vi "Test Error Propagation VITester Verify.vi"(8 "error in":errorcluster, 11 "Error.Tests in":refnum<class "Error.Propagation.Tests.lvclass">) -> (0 "error out":errorcluster, 3 "Error.Tests out":refnum<class "Error.Propagation.Tests.lvclass">)   [LabVIEW 2026, in "Error.Propagation.Tests.lvclass"]
uses:
  Error.Propagation.Tests.lvclass
  Source/Approval Tests/Options/Options.lvclass
  <vilib>/Addons/_JKI Toolkits/VI Tester/TestCase.llb/TestCase.lvclass
  Source/Approval Tests/Options/Options.lvclass/Options.ctl
  Source/Approval Tests/Naming Data/Naming Data.lvclass/Naming Data.ctl
  020b3fef-1487-42c6-8763-2b116f719ab6.vi
  020b3fef-1487-42c6-8763-2b116f719ab6.vi/ef028380-787c-4fa5-86c8-b0b7860ce2dc.vi
  Source/Approval Tests/Replace if Empty.vi
  Source/Approval Tests/Update Test Name if Not Defined.vi
  Source/Approval Tests/Verify Core.vi
  020b3fef-1487-42c6-8763-2b116f719ab6.vi/ef028380-787c-4fa5-86c8-b0b7860ce2dc.vi/93c5622b-9fb7-41e0-8c76-3fde37e94e34.vi
  Source/Approval Tests/Options/Read Scrubber.vi
  Source/Approval Tests/Naming Data/Read Test VI Name.vi
  Source/Approval Tests/Naming Data/Write Test VI Name.vi
  Source/Approval Tests/Options/Read Namer.vi
  Source/Approval Tests/Options/Read Naming Data.vi
  Source/Approval Tests/Options/Read Reporter.vi
  Source/Approval Tests/Options/Read Text Comparator.vi
  020b3fef-1487-42c6-8763-2b116f719ab6.vi/ef028380-787c-4fa5-86c8-b0b7860ce2dc.vi/93c5622b-9fb7-41e0-8c76-3fde37e94e34.vi/04cb982b-2eda-40d0-8d7e-90f8e0b569b2.vi
  Source/Approval Tests/Options/Add Label to Namer.vi
  Source/Approval Tests/conv EOL.vi
  <vilib>/Utility/libraryn.llb/Check if File or Folder Exists.vi
  Source/Approval Tests/Reporter/Report.vi
  <vilib>/addons/_JKI Toolkits/Caraya/classes/Assert/Assert True.vi
  <vilib>/addons/_JKI Toolkits/Caraya/classes/Assert/Assert Equal Value and Type_Variant.vi
  Source/Approval Tests/Scrubber/Scrubber.lvclass
  Source/Approval Tests/Namer/Namer.lvclass
  Source/Approval Tests/Naming Data/Naming Data.lvclass
  Source/Approval Tests/Reporter/Reporter.lvclass
  Source/Approval Tests/Text Comparator/Text Comparator.lvclass
  <vilib>/addons/_JKI Toolkits/Caraya/classes/Test/Test.lvclass
  <vilib>/addons/_JKI Toolkits/Caraya/classes/Assert/Assert.lvclass
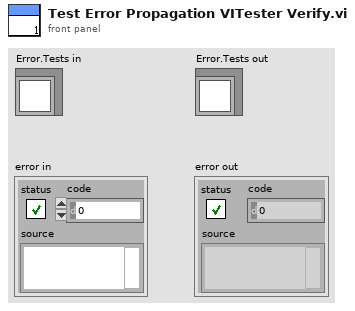
[diagram p1: front panel]
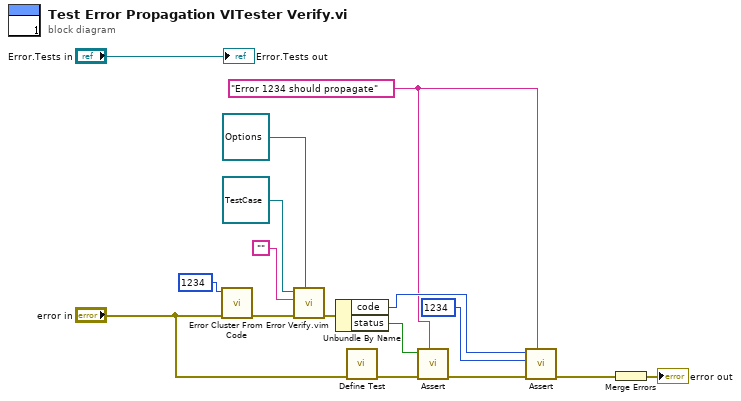
[diagram p0: block diagram]
diagram:
  w3 = "Error 1234 should propagate" ("Label (VI Title)")
  n1 = call <vilib>:"Error Cluster From Error Code.vi"("error in (no error)"="error in", "error code (0)"=1234) -> ("error out"=w13:errorcluster)  [unwired: 7 in]
  n2 = call "Verify.vim"("Options"=refnum<class "Options.lvclass"> refnum, "error in"=w13, "Test Data"="", "TestCase in"=refnum<class "TestCase.lvclass"> refnum) -> ("error out"=w12:errorcluster)  [unwired: 6 in, 1 out]
  n3 = Unbundle By Name(w12) -> ("code"=w5:i32, "status"=w6:bool)
  n4 = call <vilib>:"Define Test.vi"("error in (no error)"="error in") -> ("error out"=w16:errorcluster)  [unwired: 9 in, 1 out]
  n5 = call-poly <vilib>:"Assert.vi"("Label"=w3, "error in (no error)"=w16, "True?"=w6) -> ("error out"=w11:errorcluster)  [unwired: 7 in, 1 out]
  n6 = call-poly <vilib>:"Assert.vi"("Label"=w3, "error in (no error)"=w11, "Actual"=1234 ("error code (1)"), "Expected"=w5) -> ("error out"=w10:errorcluster)  [unwired: 6 in, 1 out]
  n7 = Merge Errors(w10) -> (→"error out":errorcluster)
  "Error.Tests out" <- "Error.Tests in"
